vi "create_spiral.vi"(7 "angular shift":dbl, 8 "error in (no error)":errorcluster, 9 "no. of points in spiral":i32, 10 "offset":refnum<class "SpaceVector.lvclass">, 11 "TrajectoryDL121017Hopping in":refnum<class "TrajectoryDL121017Hopping.lvclass">) -> (0 "error out":errorcluster, 2 "spiral":refnum<class "SpaceVector.lvclass">[](array[class]), 3 "TrajectoryDL121017Hopping out":refnum<class "TrajectoryDL121017Hopping.lvclass">)   [LabVIEW 2010, in "TrajectoryDL121017Hopping.lvclass"]
doc: "Creates the coordinates for a uncaging spiral for one single ROI."
uses:
  TrajectoryDL121017Hopping.lvclass
  common/classes/SpaceVector/SpaceVector/SpaceVector.lvclass
  <vilib>/Native 3D Graph/xcontrol/3DPC_SurfacePlot.xctl
  TrajectoryDL121017Hopping.lvclass/TrajectoryDL121017Hopping.ctl
panel:
  out "3D Graph 2":refnum<class "Base Datatype.lvclass">[](xcontrol)
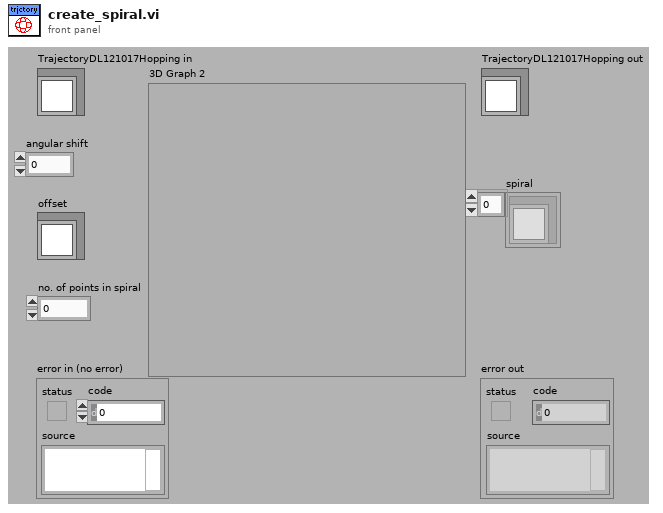
[diagram p1: front panel]
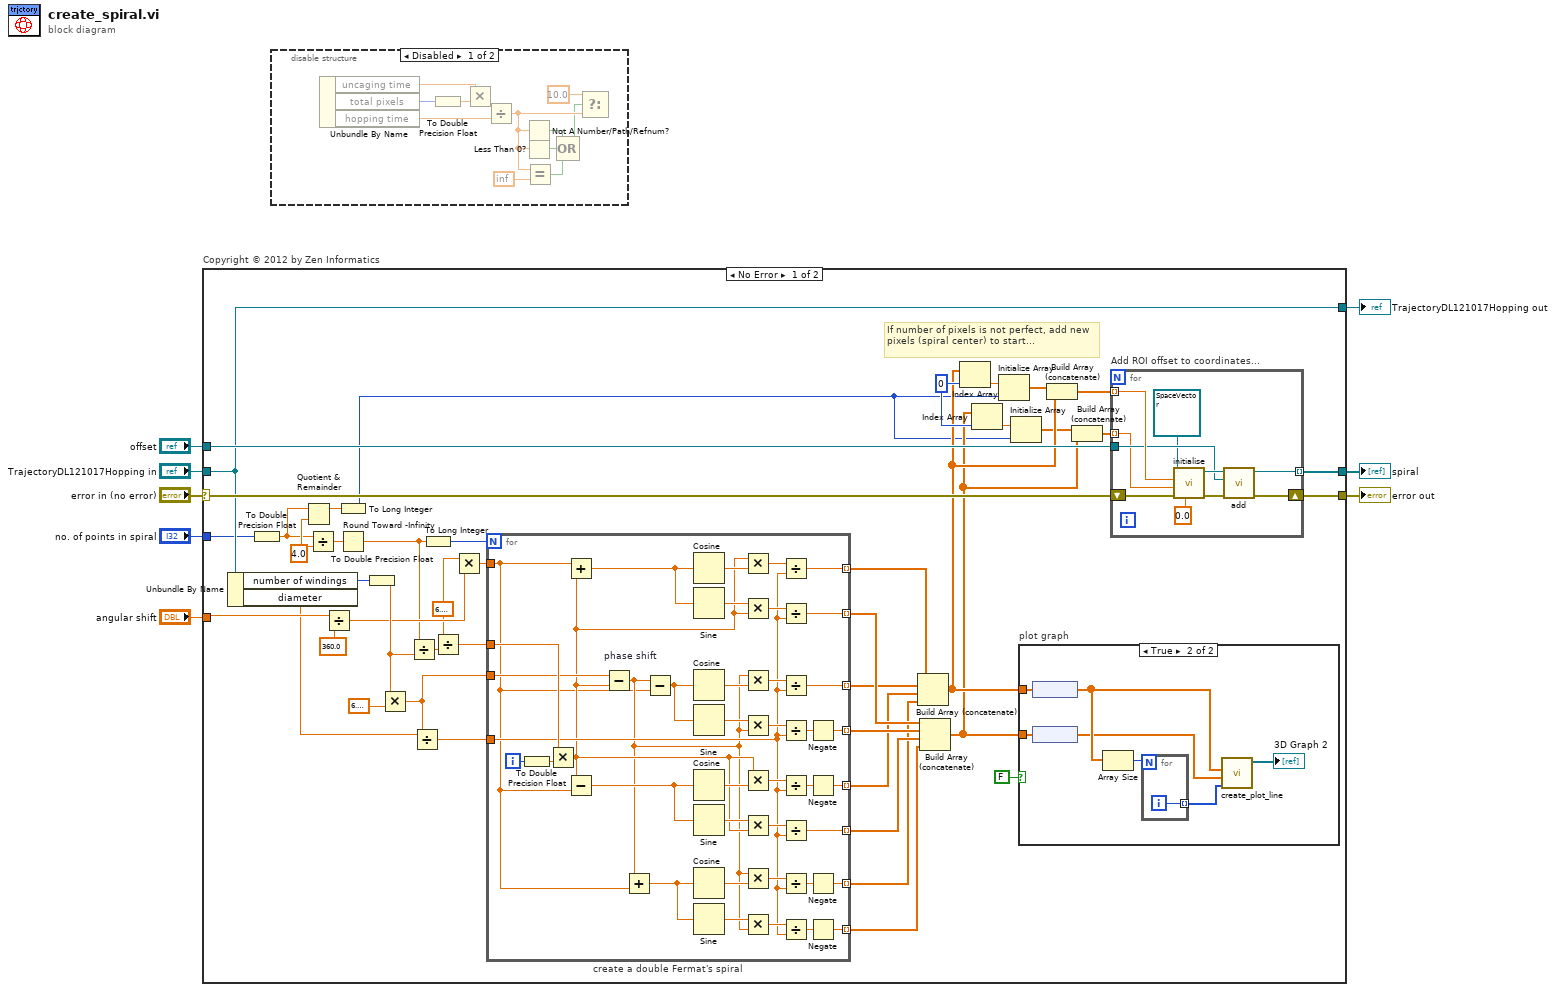
[diagram p0: block diagram]
diagram:
  n1 = case "Copyright © 2012 by Zen Informatics" shown="No Error" "error in (no error)" {
    selector: "error in (no error)" -> [w30 w112]
    tunnel: [w50 w112] -> w7
    tunnel: [w29 w111] -> w5
    tunnel: "TrajectoryDL121017Hopping in" -> [w29 w111]
    tunnel: [w49 _] -> w4
    tunnel: "offset" -> [w48 _]
    tunnel: "angular shift" -> [w34 _]
    tunnel: "no. of points in spiral" -> [w25 _]
    frame No Error {
      w16 = 0 ("index")
      w21 = 4.0 ("y")
      w26 = 6.283185307179586
      # "If number of pixels is not perfect, add new pixels (spiral center) to start..."
      n2 = Unbundle By Name(w29) -> ("number of windings"=w27:i32, "diameter"=w28:dbl[unit])
      n3 = To Double Precision Float(number=w25) -> (double precision float=w20:dbl)
      n4 = Quotient & Remainder(x=w20, y=w21) -> (x-y*floor(x/y)=w19:dbl)  [unwired: 1 out]
      n5 = Divide(x=w20, y=w21) -> (x/y=w24:dbl)
      n6 = Divide(x=w34, y=360.0) -> (x/y=w32:dbl)
      n7 = To Long Integer(number=w19) -> (32bit integer=w9:i32)
      n8 = Round Toward -Infinity(1:w24) -> (0:w23:dbl)
      n9 = To Double Precision Float(number=w27) -> (double precision float=w35:dbl)
      n10 = Multiply(x=w35, y=6.283185307179586) -> (x*y=w43:dbl)
      n11 = Divide(x=w23, y=w35) -> (x/y=w51:dbl)
      n12 = Divide(x=w43, y=w28) -> (x/y=w46:dbl[unit])
      n13 = To Long Integer(number=w23) -> (32bit integer=w22:i32)
      n14 = Divide(x=w26, y=w51) -> (x/y=w47:dbl)
      n15 = Multiply(x=w26, y=w32) -> (x*y=w40:dbl)
      n16 = for "create a double Fermat's spiral" {
        N: w22 -> [_]
        tunnel: w47 -> [w100]
        tunnel: [w84] -> w42 mode=indexing
        tunnel: [w93] -> w45 mode=indexing
        tunnel: w46 -> [w72]
        tunnel: w40 -> [w61]
        tunnel: [w86] -> w41 mode=indexing
        tunnel: [w85] -> w44 mode=indexing
        tunnel: w43 -> [w87]
        tunnel: [w77] -> w39 mode=indexing
        tunnel: [w79] -> w38 mode=indexing
        tunnel: [w67] -> w37 mode=indexing
        tunnel: [w66] -> w36 mode=indexing
        i -> [w94]
        n17 = To Double Precision Float(number=w94) -> (double precision float=w95:dbl)
        n18 = Multiply(x=w100, y=w95) -> (x*y=w70:dbl)
        n19 = Add ("add rotation")(x=w61, y=w70) -> (x+y=w65:dbl)
        n20 = Subtract(x=w70, y=w61) -> (x-y=w71:dbl)
        n21 = Subtract "phase shift"(x=w87, y=w70) -> (x-y=w63:dbl)
        n22 = Add(x=w63, y=w61) -> (x+y=w62:dbl)
        n23 = Subtract(x=w63, y=w61) -> (x-y=w64:dbl)
        n24 = Cosine(x=w65) -> (cos(x)=w99:dbl)
        n25 = Sine(x=w65) -> (sin(x)=w98:dbl)
        n26 = Cosine(x=w64) -> (cos(x)=w89:dbl)
        n27 = Sine(x=w64) -> (sin(x)=w90:dbl)
        n28 = Cosine(x=w71) -> (cos(x)=w80:dbl)
        n29 = Sine(x=w71) -> (sin(x)=w81:dbl)
        n30 = Cosine(x=w62) -> (cos(x)=w76:dbl)
        n31 = Sine(x=w62) -> (sin(x)=w75:dbl)
        n32 = Multiply(x=w70, y=w99) -> (x*y=w96:dbl)
        n33 = Multiply(x=w98, y=w70) -> (x*y=w97:dbl)
        n34 = Multiply(x=w63, y=w89) -> (x*y=w92:dbl)
        n35 = Multiply(x=w90, y=w63) -> (x*y=w91:dbl)
        n36 = Multiply(x=w70, y=w80) -> (x*y=w83:dbl)
        n37 = Multiply(x=w81, y=w70) -> (x*y=w82:dbl)
        n38 = Multiply(x=w63, y=w76) -> (x*y=w73:dbl)
        n39 = Multiply(x=w75, y=w63) -> (x*y=w74:dbl)
        n40 = Divide(x=w96, y=w72) -> (x/y=w84:dbl[unit])
        n41 = Divide(x=w97, y=w72) -> (x/y=w93:dbl[unit])
        n42 = Divide(x=w92, y=w72) -> (x/y=w86:dbl[unit])
        n43 = Divide(x=w91, y=w72) -> (x/y=w88:dbl[unit])
        n44 = Divide(x=w83, y=w72) -> (x/y=w78:dbl[unit])
        n45 = Divide(x=w82, y=w72) -> (x/y=w79:dbl[unit])
        n46 = Divide(x=w73, y=w72) -> (x/y=w69:dbl[unit])
        n47 = Divide(x=w74, y=w72) -> (x/y=w68:dbl[unit])
        n48 = Negate(x=w88) -> (-x=w85:dbl[unit])
        n49 = Negate(x=w78) -> (-x=w77:dbl[unit])
        n50 = Negate(x=w69) -> (-x=w67:dbl[unit])
        n51 = Negate(x=w68) -> (-x=w66:dbl[unit])
      }
      n52 = Build Array (concatenate)(w42, w41, w39, w37) -> (w14:dbl[unit][])
      n53 = Build Array (concatenate)(w45, w44, w38, w36) -> (w12:dbl[unit][])
      n54 = Index Array(array=w14, index=w16) -> (element=w18:dbl[unit])
      n55 = Index Array(array=w12, index=w16) -> (element=w17:dbl[unit])
      n56 = Initialize Array(w18, w9) -> (w15:dbl[unit][])
      n57 = Initialize Array(w17, w9) -> (w11:dbl[unit][])
      n58 = case "plot graph" shown="True" FALSE {
        tunnel: w14 -> [_ w59]
        tunnel: w12 -> [_ w58]
        frame False {
        }
        frame True {
          n59 = node(w59) -> (w54:dbl[])
          n60 = node(w58) -> (w53:dbl[])
          n61 = Array Size(array=w54) -> (size(s)=w56:i32)
          n62 = for {
            N: w56 -> [_]
            tunnel: [w60] -> w57 mode=indexing
            i -> [w60]
          }
          n63 = call <vilib>:"create_plot_line.vi"("z vector"=w57, "y vector"=w53, "x vector"=w54) -> ("plots out"=→"3D Graph 2":refnum<class "Base Datatype.lvclass">[])  [unwired: 2 in, 6 out]
        }
      }
      n64 = Build Array (concatenate)(w15, w14) -> (w13:dbl[unit][])
      n65 = Build Array (concatenate)(w11, w12) -> (w10:dbl[unit][])
      n66 = for "Add ROI offset to coordinates..." {
        tunnel: w48 -> [w106]
        tunnel: w13 -> [w109] mode=indexing
        shift-right: [w103] -> w50
        shift-left: w30 -> [w110]
        tunnel: [w104] -> w49 mode=indexing
        tunnel: w10 -> [w101] mode=indexing
        n67 = call "initialise.vi"("z"=dbl[unit] 0.0, "error in (no error)"=w110, "y"=w101, "x"=w109, "SpaceVector in"=refnum<class "SpaceVector.lvclass"> refnum) -> ("error out"=w108:errorcluster, "SpaceVector out"=w107:refnum<class "SpaceVector.lvclass">)  [unwired: 5 in]
        n68 = call "add.vi"("error in (no error)"=w108, "vector to be added"=w106, "SpaceVector in"=w107) -> ("error out"=w103:errorcluster, "SpaceVector out"=w104:refnum<class "SpaceVector.lvclass">)  [unwired: 7 in]
      }
    }
    frame Error {
    }
  }
  "error out" <- w7
  "TrajectoryDL121017Hopping out" <- w5
  "spiral" <- w4
  n69 = disable-structure shown="Disabled" {
    frame Disabled {
      n70 = Unbundle By Name() -> ("uncaging time"=w113:dbl[unit], "total pixels"=w114:i32, "hopping time"=w116:dbl[unit])  [unwired: 1 in]
      n71 = To Double Precision Float(number=w114) -> (double precision float=w115:dbl)
      n72 = Multiply(x=w113, y=w115) -> ()  [unwired: 1 out]
      n73 = Divide(y=w116) -> (x/y=w121:dbl)  [unwired: 1 in]
      n74 = Not A Number/Path/Refnum?(number/path/refnum=w121) -> (NaN/Path/Refnum?=w119:bool)
      n75 = Less Than 0?(x=w121) -> (x < 0?=w118:bool)
      n76 = Equal?(x=w121, y=inf) -> (x = y?=w123:bool)
      n77 = Compound Arithmetic op=OR(w119, w118, w123) -> (w120:bool)
      n78 = Select(t=10.0, s=w120, f=w121) -> ()  [unwired: 1 out]
    }
    frame Enabled {
    }
  }
